vi "oa_TV Average Angle Intervals (NChan).vi"(6 "revulotion index":i32[](array[numeric]), 7 "reset? (F)":bool, 8 "error in (no error)":errorcluster, 9 "pulse/revolution":i32[](array[numeric]), 10 "RPM":cluster{dbl[]}[](array[cluster]), 11 "time index":cluster{dbl[]}[](array[cluster])) -> (0 "error out":errorcluster, 3 "angle intervals":cluster{"angle intervals":dbl[]}[](array[cluster]))   [LabVIEW 2017, in "SoundVib_Torsional.lvlib"]
uses:
  <vilib>/addons/Sound and Vibration/Order Analysis/Torsional Vibration/SoundVib_Torsional.lvlib
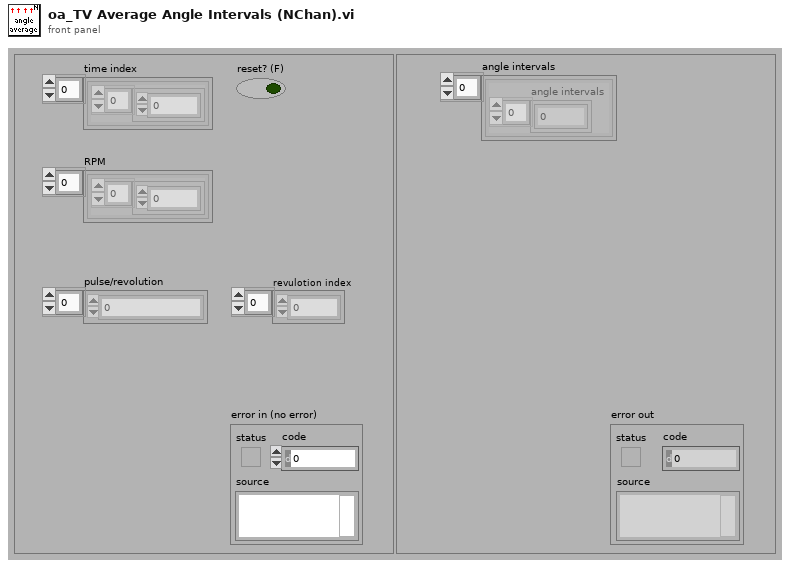
[diagram p1: front panel]
types:
  T1 = enum16{"Exponential average", "Moving average", "Current"}
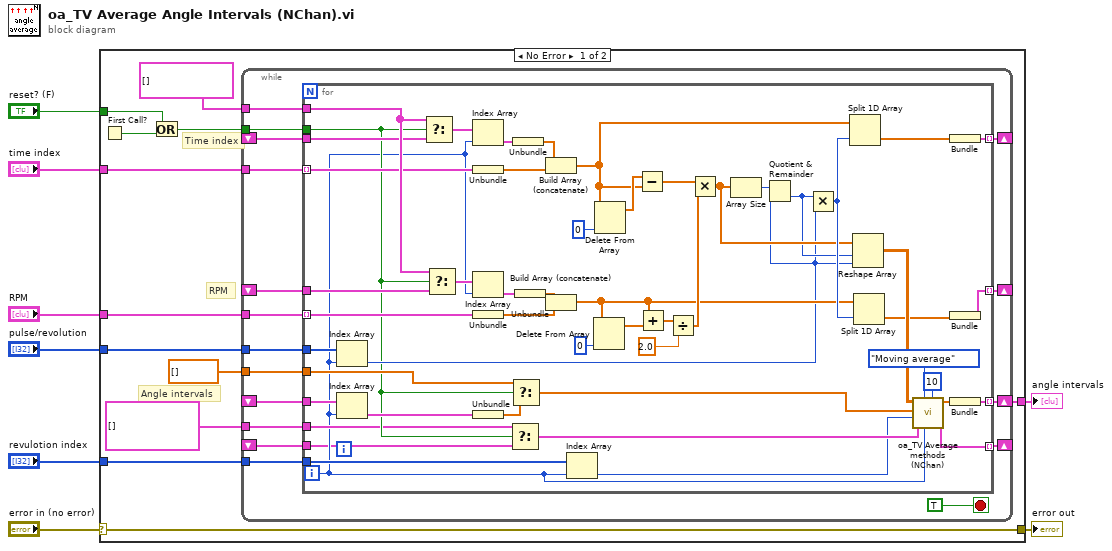
[diagram p0: block diagram]
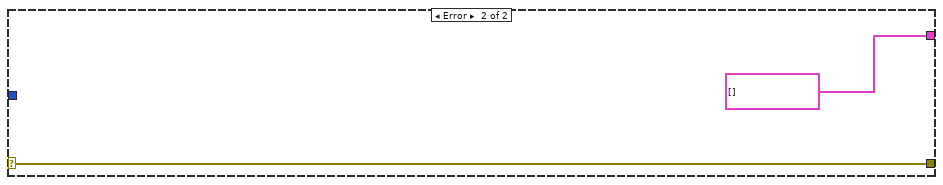
[diagram p2: hidden frame]
diagram:
  n1 = case shown="No Error" "error in (no error)" {
    selector: "error in (no error)" -> [w18 w90]
    tunnel: "RPM" -> [w14 _]
    tunnel: "pulse/revolution" -> [w20 _]
    tunnel: "revulotion index" -> [w19 _]
    tunnel: [w17 cluster{"Angle intervals":dbl[]}[] []] -> w2
    tunnel: [w18 w90] -> w7
    tunnel: "time index" -> [w13 _]
    tunnel: "reset? (F)" -> [w10 _]
    frame No Error {
      # "Angle intervals"
      # "RPM"
      # "Time index"
      n2 = First Call?() -> (First Call?: T/F=w16:bool)
      n3 = Or(x=w10, y=w16) -> (x .or. y?=w15:bool)
      n4 = while {
        tunnel: w14 -> [w35]
        shift-right: [w24] -> _
        shift-left: _ -> [w37]
        shift-right: [w34] -> _
        shift-left: _ -> [w36]
        tunnel: w15 -> [w29]
        tunnel: cluster{dbl[]}[] [] -> [w31]
        tunnel: w20 -> [w33]
        shift-right: [w28] -> w17
        shift-left: _ -> [w30]
        tunnel: w19 -> [w27]
        tunnel: w13 -> [w26]
        tunnel: dbl[] [] ("t") -> [w25]
        shift-right: [w22] -> _
        shift-left: _ -> [w21]
        tunnel: cluster{dbl[][]}[] [] -> [w23]
        stop <- TRUE stop-if-true
        n5 = for {
          tunnel: w37 -> [w57]
          tunnel: w36 -> [w55]
          tunnel: w26 -> [w59] mode=indexing
          tunnel: w35 -> [w63] mode=indexing
          tunnel: [w51] -> w24 mode=indexing
          tunnel: [w45] -> w34 mode=indexing
          tunnel: w33 -> [w61]
          tunnel: w31 -> [w75]
          tunnel: w30 -> [w67]
          tunnel: w29 -> [w44]
          tunnel: [w68] -> w28 mode=indexing
          tunnel: w27 -> [w64]
          tunnel: w25 -> [w53]
          tunnel: w23 -> [w43]
          tunnel: [w39] -> w22 mode=indexing
          tunnel: w21 -> [w38]
          i -> [w40]
          n6 = Index Array(array=w61, index=w40) -> (element=w60:i32)
          n7 = Index Array(array=w67, index=w40) -> (element=w66:cluster{"Angle intervals":dbl[]})
          n8 = Select(t=w75, s=w44, f=w57) -> (s? t:f=w56:cluster{dbl[]}[])
          n9 = Select(t=w75, s=w44, f=w55) -> (s? t:f=w54:cluster{dbl[]}[])
          n10 = Index Array(array=w56, index=w40) -> (element=w50:cluster{dbl[]})
          n11 = Unbundle(w59) -> (w58:dbl[])
          n12 = Index Array(array=w54, index=w40) -> (element=w48:cluster{dbl[]})
          n13 = Unbundle(w63) -> (w62:dbl[])
          n14 = Unbundle(w66) -> ("Angle intervals"=w65:dbl[])
          n15 = Select(t=w43, s=w44, f=w38) -> (s? t:f=w42:cluster{dbl[][]}[])
          n16 = Select(t=w53, s=w44, f=w65) -> (s? t:f=w72:dbl[])
          n17 = Unbundle(w50) -> (w49:dbl[])
          n18 = Unbundle(w48) -> (w47:dbl[])
          n19 = Build Array (concatenate)(w49, w58) -> (w80:dbl[])
          n20 = Build Array (concatenate)(w47, w62) -> (w74:dbl[])
          n21 = Index Array(array=w64, index=w40) -> (element=w41:i32)
          n22 = Delete From Array(array=w74, index=0) -> (array with subset deleted=w81:dbl[])  [unwired: 1 in, 1 out]
          n23 = Delete From Array(array=w80, index=0) -> (array with subset deleted=w82:dbl[])  [unwired: 1 in, 1 out]
          n24 = Subtract(x=w82, y=w80) -> (x-y=w84:dbl[])
          n25 = Add(x=w74, y=w81) -> (x+y=w86:dbl[])
          n26 = Divide(x=w86, y=2.0) -> (x/y=w79:dbl[])
          n27 = Multiply(x=w84, y=w79) -> (x*y=w77:dbl[])
          n28 = Array Size(array=w77) -> (size(s)=w83:i32)
          n29 = Quotient & Remainder(x=w83, y=w60) -> (floor(x/y)=w76:i32)  [unwired: 1 out]
          n30 = Multiply(x=w76, y=w60) -> (x*y=w78:i32)
          n31 = Split 1D Array(array=w80, index=w78) -> (second subarray=w52:dbl[])  [unwired: 1 out]
          n32 = Reshape Array(w77, w76, w60) -> (w73:dbl[][])
          n33 = Split 1D Array(array=w74, index=w78) -> (second subarray=w46:dbl[])  [unwired: 1 out]
          n34 = call <vilib>:"oa_TV Average methods (NChan).vi"("Window size"=i16 10, "channel index"=w40, "Enum"=T1."Moving average", "previous date"=w42, "Revulotion index"=w41, "Angle intervals"=w72, "Array"=w73) -> ("Previous data"=w39:cluster{dbl[][]}, "Angle intervals"=w69:dbl[])  [unwired: 3 in]
          n35 = Bundle(w52) -> (w51:cluster{dbl[]})  [unwired: 1 in]
          n36 = Bundle(w46) -> (w45:cluster{dbl[]})  [unwired: 1 in]
          n37 = Bundle("Angle intervals"=w69) -> (w68:cluster{"Angle intervals":dbl[]})  [unwired: 1 in]
        }
      }
    }
    frame Error {
    }
  }
  "error out" <- w7
  "angle intervals" <- w2
